vi "TSM SSC DCPower Initiate.vi"(0 "DCPower TSM in":T1, 11 "error in":errorcluster) -> (4 "DCPower TSM out":T1, 15 "error out":errorcluster)   [LabVIEW 2019]
doc: "Starts generation or acquisition, causing the NI-DCPower sessions to leave the Uncommitted state or Committed state and enter the Running state."
uses:
  TSM/TSM SSC DCPower.ctl
  <vilib>/NI_TestStand_SemiconductorModule/NI_TestStand_Semiconductor_Module.lvlibp/PinMap/PinQueryContext/MultiplePinMultipleSessionQueryContext/MultiplePinMultipleSessionQueryContext.lvclass
  SSC DCPower/SSC DCPower.ctl
  Shared SubVIs/TSM Pin Abstraction/TSM Pin Information.ctl
  Shared SubVIs/TSM Pin Abstraction/TSM Pin Type Identifier.ctl
  Shared SubVIs/TSM Pin Abstraction/TSM Expanded Pin Information.ctl
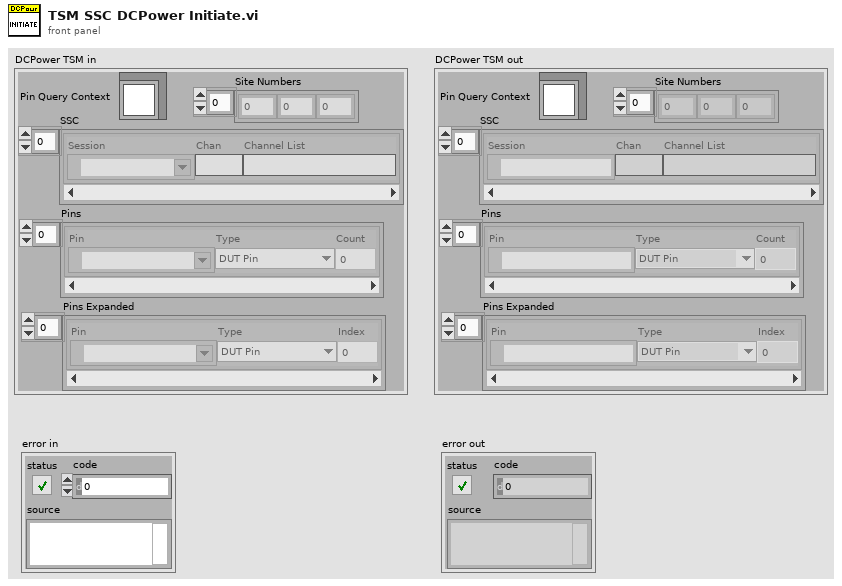
[diagram p1: front panel]
types:
  T1 = typedef "TSM SSC DCPower.ctl" = cluster{"Pin Query Context":refnum<class "MultiplePinMultipleSessionQueryContext.lvclass">, "SSC":T2[], "Site Numbers":i32[], "Pins":T3[], "Pins Expanded":T5[]}
  T2 = typedef "SSC DCPower.ctl" = cluster{"Session":refnum<k15>, "Chan":string, "Channel List":string}
  T3 = typedef "TSM Pin Information.ctl" = cluster{"Pin":tag, "Type":T4, "Count":i32}
  T4 = typedef "TSM Pin Type Identifier.ctl" = enum8{"DUT Pin", "System Pin", "Pin Group", "Not Determined"}
  T5 = typedef "TSM Expanded Pin Information.ctl" = cluster{"Pin":tag, "Type":T4, "Index":i32}
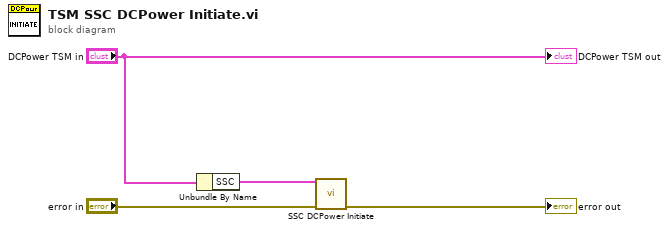
[diagram p0: block diagram]
diagram:
  n1 = Unbundle By Name("DCPower TSM in") -> ("SSC"=w1:T2[])
  n2 = call "SSC DCPower Initiate.vi"("DCPower SSC in"=w1, "error in"="error in") -> ("error out"=→"error out":errorcluster)  [unwired: 12 in, 1 out]
  "DCPower TSM out" <- "DCPower TSM in"
